vi "MSScript_Act_ExtractHeader.vi"(8 "error in (no error)":errorcluster, 11 "MSScript in":refnum<class "MSScript.lvclass">) -> (0 "error out":errorcluster, 3 "MSScript out":refnum<class "MSScript.lvclass">)   [LabVIEW 2018, in "MSScript.lvclass"]
uses:
  MSScript.lvclass
  MSScript.lvclass/MSScript.ctl
  MSScript_Error_(6003)HeaderLost.vi
  MSScript_Error_(6001)VariableError.vi
  MSScript_Error_(6002)UndefinedSentence.vi
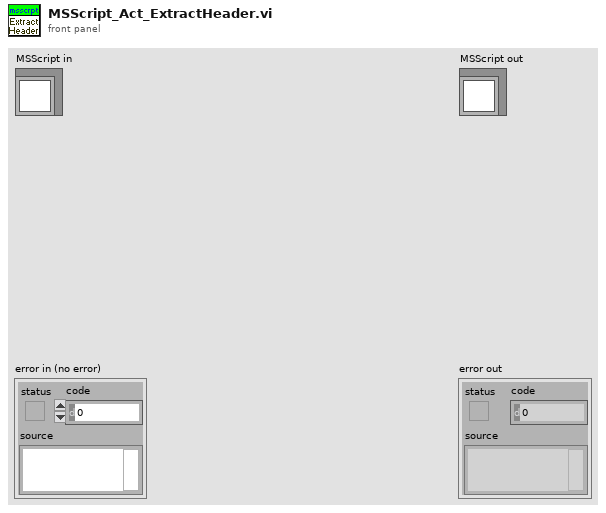
[diagram p1: front panel]
types:
  T1 = cluster{"Colour":u32, "Italic":bool, "Bold":bool}
  T2 = cluster{"Type":string, "NAME":cluster{"STR":string, "Start":i32}, "PARAMs":cluster{"STR":string, "Start":i32}[]}[]
  T3 = cluster{"Type":string, "NAME":cluster{"STR":string, "Start":i32}, "PARAMs":cluster{"STR":string, "Start":i32}[]}
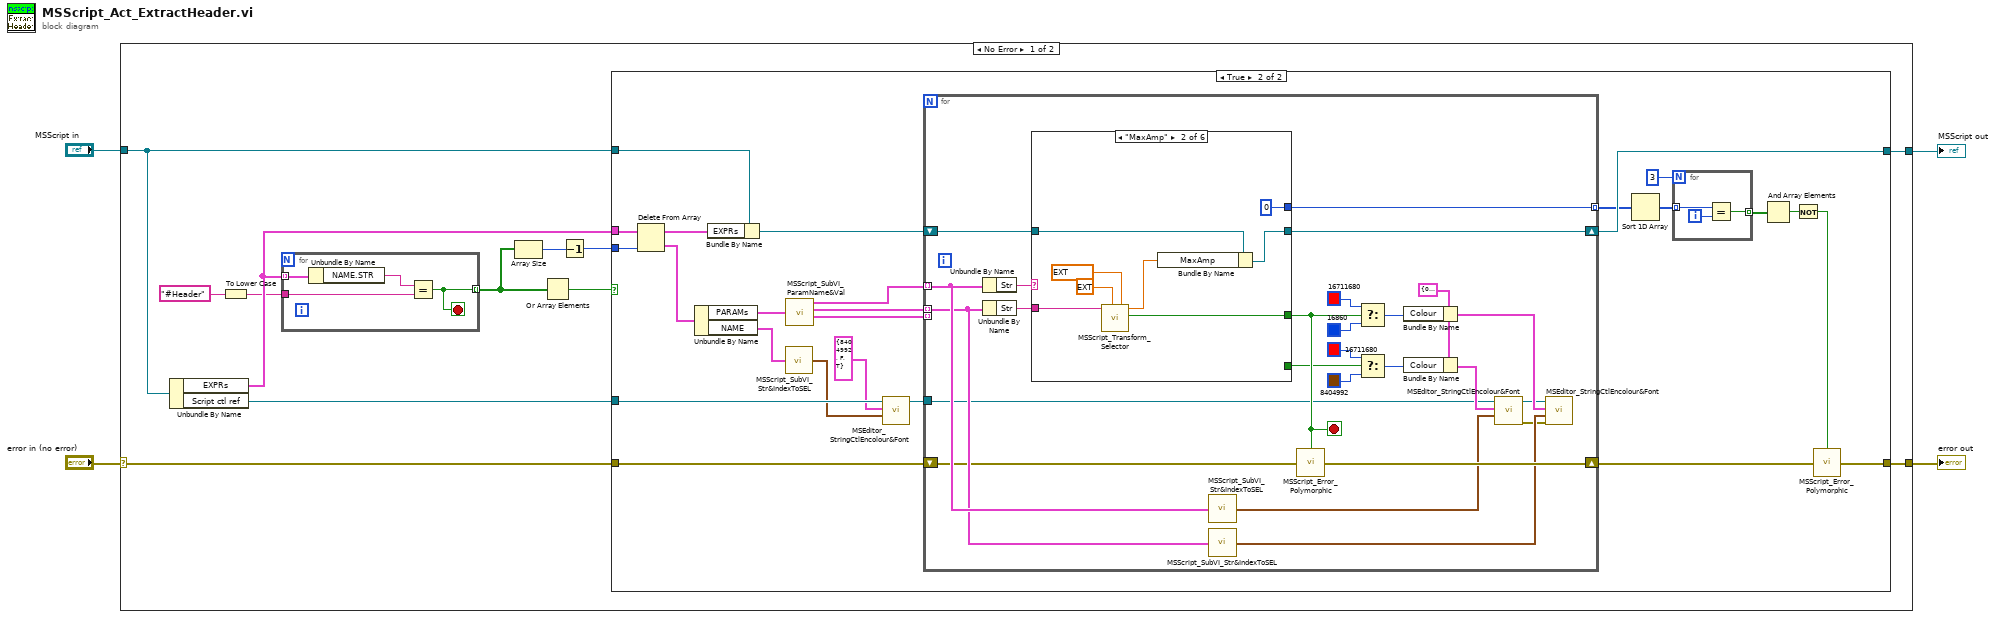
[diagram p0: block diagram]
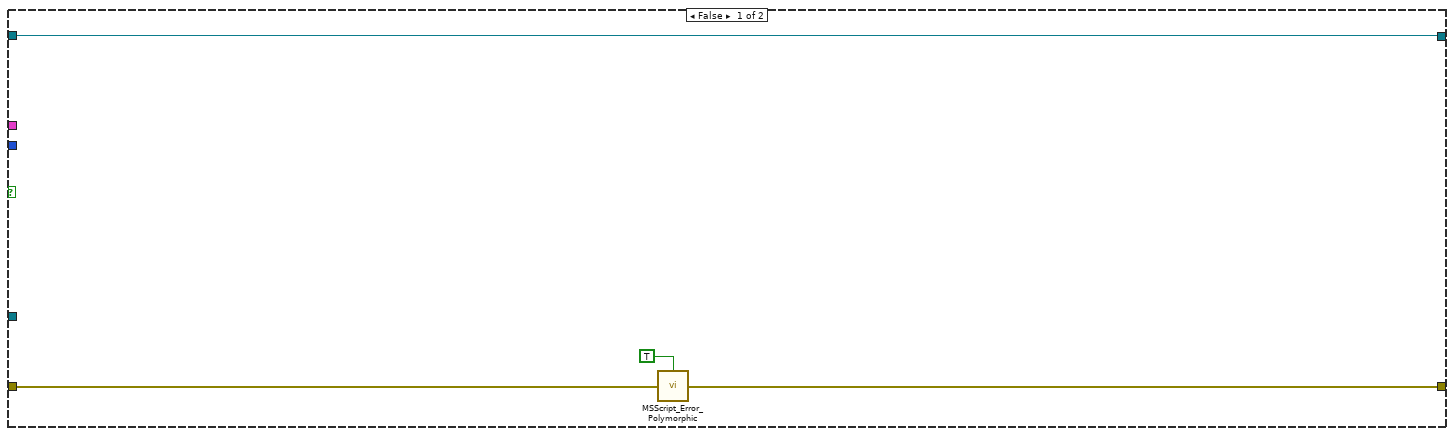
[diagram p2: hidden frame]
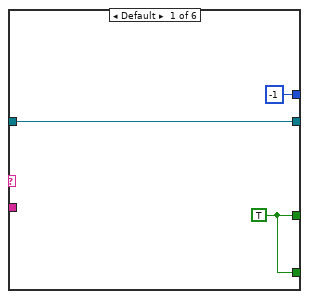
[diagram p3: hidden frame]
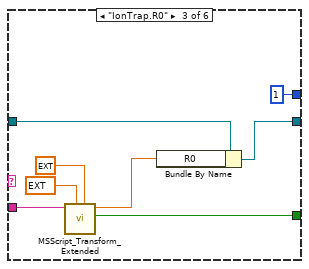
[diagram p4: hidden frame]
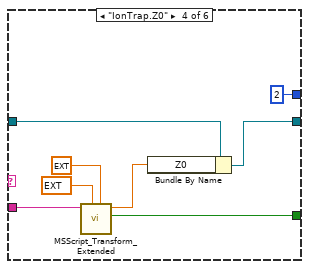
[diagram p5: hidden frame]
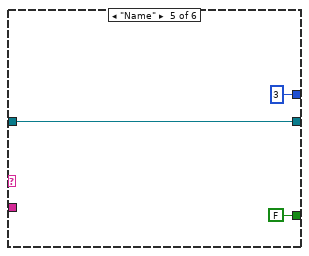
[diagram p6: hidden frame]
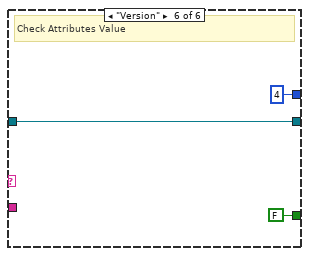
[diagram p7: hidden frame]
diagram:
  n1 = case shown="No Error" "error in (no error)" {
    selector: "error in (no error)" -> [w13 w112]
    tunnel: [w11 w112] -> w3
    tunnel: [w12 w111] -> w1
    tunnel: "MSScript in" -> [w15 w111]
    frame No Error {
      n2 = Unbundle By Name(w15) -> ("EXPRs"=w16:T2, "Script ctl ref"=w14:refnum<vi>)
      n3 = To Lower Case(string="#Header") -> (all lower case string=w9:string)
      n4 = for {
        tunnel: w16 -> [w110] mode=indexing
        tunnel: [w107] -> w7 mode=indexing
        tunnel: w9 -> [w109]
        stop <- w107 stop-if-true
        n5 = Unbundle By Name(w110) -> ("NAME.STR"=w108:string)
        n6 = Equal?(x=w108, y=w109) -> (x = y?=w107:bool)
      }
      n7 = Array Size(array=w7) -> (size(s)=w6:i32)
      n8 = Or Array Elements(Boolean array=w7) -> (logical OR=w8:bool)
      n9 = Decrement(x=w6) -> (x-1=w5:i32)
      n10 = case shown="True" w8 {
        tunnel: w16 -> [_ w45]
        tunnel: w15 -> [w20 w29]
        tunnel: w14 -> [_ w36]
        tunnel: w13 -> [w19 w39]
        tunnel: [w20 w32] -> w12
        tunnel: [w18 w30] -> w11
        tunnel: w5 -> [_ w27]
        frame False {
          n11 = call-poly "MSScript_Error_Polymorphic.vi"("error in (no error)"=w19, "ErrBoolean"=TRUE) -> ("error out"=w18:errorcluster)
        }
        frame True {
          n12 = Delete From Array(array=w45, index=w27) -> (deleted portion=w43:T3, array with subset deleted=w44:T2)  [unwired: 1 in]
          n13 = Unbundle By Name(w43) -> ("PARAMs"=w42:cluster{"STR":string, "Start":i32}[], "NAME"=w38:cluster{"STR":string, "Start":i32})
          n14 = Bundle By Name(cluster=w29, "EXPRs"=w44) -> (w28:refnum<class "MSScript.lvclass">)
          n15 = call "MSScript_SubVI_Str&IndexToSEL.vi"("Name string"=w38) -> ("SEL"=w35:cluster{"Start":u32, "End":u32}[])
          n16 = call "MSScript_SubVI_ParamName&Val.vi"("PARAMs"=w42) -> ("PARAM.NAMEs"=w41:cluster{"Str":string, "Start":i32}[], "PARAM.VALs"=w40:cluster{"Str":string, "Start":i32}[], "PARAM.EqualSign"=w33:cluster{"Str":string, "Start":i32}[])  [unwired: 4 in, 1 out]
          n17 = call "MSEditor_StringCtlEncolour&Font.vi"("SELs"=w35, "TextProperties"=T1 {"Colour"=8404992, "Italic"=FALSE, "Bold"=TRUE}, "String ctl ref"=w36) -> ("String ctl ref out"=w37:refnum<vi>)  [unwired: 7 in, 1 out]
          n18 = for {
            shift-right: [w70] -> w32
            shift-left: w28 -> [w72]
            tunnel: w41 -> [w63] mode=indexing
            tunnel: w40 -> [w61] mode=indexing
            tunnel: w37 -> [w50]
            tunnel: w33 -> [_] mode=indexing
            shift-right: [w65] -> w31
            shift-left: w39 -> [w60]
            tunnel: [w49] -> w23 mode=indexing
            stop <- w64 stop-if-true
            w52 = T1 {"Colour"=0, "Italic"=FALSE, "Bold"=FALSE} ("TextProperties")
            n19 = Unbundle By Name(w63) -> ("Str"=w73:string)
            n20 = Unbundle By Name(w61) -> ("Str"=w71:string)
            n21 = case shown="\"MaxAmp\"" w73 {
              tunnel: w72 -> [w76 w79 w88 w96 w103 w106]
              tunnel: w71 -> [_ w83 w92 w100 _ _]
              tunnel: [w76 w84 w87 w94 w103 w106] -> w70
              tunnel: [w75 w80 w86 w95 FALSE ("Value Error?") FALSE ("Value Error?")] -> w64
              tunnel: [w75 _ _ _ _ _] -> w56
              tunnel: [-1 0 1 2 3 4] -> w49
              frame Default {
                w75 = TRUE ("Value Error?")
              }
              frame "MaxAmp" {
                n22 = call-poly "MSScript_Transform_Selector.vi"("upper limit (Inf)"=ext 100000.0 ("upper limit"), "lower limit (-Inf)"=ext 0.0 ("lower limit"), "Check_Str"=w83) -> ("Value Error?"=w80:bool, "Value Output"=w78:ext)  [unwired: 6 in, 1 out]
                n23 = Bundle By Name(cluster=w79, "MaxAmp"=w78) -> (w84:refnum<class "MSScript.lvclass">)
              }
              frame "IonTrap.R0" {
                n24 = call "MSScript_Transform_Extended.vi"("upper limit (Inf)"=ext 20.0 ("upper limit"), "lower limit (-Inf)"=ext 0.01 ("lower limit"), "Check_Str"=w92) -> ("Value Error?"=w86:bool, "Value Output"=w89:ext)  [unwired: 6 in, 1 out]
                n25 = Bundle By Name(cluster=w88, "R0"=w89) -> (w87:refnum<class "MSScript.lvclass">)
              }
              frame "IonTrap.Z0" {
                n26 = call "MSScript_Transform_Extended.vi"("upper limit (Inf)"=ext 20.0 ("upper limit"), "lower limit (-Inf)"=ext 0.01 ("lower limit"), "Check_Str"=w100) -> ("Value Error?"=w95:bool, "Value Output"=w97:ext)  [unwired: 6 in, 1 out]
                n27 = Bundle By Name(cluster=w96, "Z0"=w97) -> (w94:refnum<class "MSScript.lvclass">)
              }
              frame "Name" {
              }
              frame "Version" {
                # "Check Attributes Value"
              }
            }
            n28 = call "MSScript_SubVI_Str&IndexToSEL.vi"("Name string"=w63) -> ("SEL"=w59:cluster{"Start":u32, "End":u32}[])
            n29 = call "MSScript_SubVI_Str&IndexToSEL.vi"("Name string"=w61) -> ("SEL"=w62:cluster{"Start":u32, "End":u32}[])
            n30 = call-poly "MSScript_Error_Polymorphic.vi"("error in (no error)"=w60, "ErrBoolean"=w64) -> ("error out"=w65:errorcluster)
            n31 = Select(t=u32 16711680, s=w64, f=u32 16860) -> (s? t:f=w69:u32)
            n32 = Select(t=u32 16711680, s=w56, f=u32 8404992 ("Colour")) -> (s? t:f=w53:u32)
            n33 = Bundle By Name(cluster=w52, "Colour"=w69) -> (w68:T1)
            n34 = Bundle By Name(cluster=w52, "Colour"=w53) -> (w51:T1)
            n35 = call "MSEditor_StringCtlEncolour&Font.vi"("SELs"=w59, "TextProperties"=w51, "String ctl ref"=w50) -> ("error out"=w57:errorcluster, "String ctl ref out"=w58:refnum<vi>)  [unwired: 7 in]
            n36 = call "MSEditor_StringCtlEncolour&Font.vi"("error in (no error)"=w57, "SELs"=w62, "TextProperties"=w68, "String ctl ref"=w58) -> ()  [unwired: 6 in, 2 out]
          }
          n37 = Sort 1D Array(array=w23) -> (sorted array=w22:i32[])
          n38 = for {
            N: 3 -> [_]
            tunnel: w22 -> [w47] mode=indexing
            tunnel: [w46] -> w25 mode=indexing
            i -> [w48]
            n39 = Equal?(x=w47, y=w48) -> (x = y?=w46:bool)
          }
          n40 = And Array Elements(Boolean array=w25) -> (logical AND=w24:bool)
          n41 = Not(x=w24) -> (.not. x?=w21:bool)
          n42 = call-poly "MSScript_Error_Polymorphic.vi"("error in (no error)"=w31, "ErrBoolean"=w21) -> ("error out"=w30:errorcluster)
        }
      }
    }
    frame Error {
    }
  }
  "error out" <- w3
  "MSScript out" <- w1
